vi "set_sensor_parameters_cluster.vi"(8 "error in (no error)":errorcluster, 9 "Sensor parameters":T1, 10 "Sensor number":u8, 11 "VISA resource name":refnum<visa-resource-name>) -> (0 "error out":errorcluster, 3 "VISA resource name out":refnum<visa-resource-name>)   [LabVIEW 2018]
doc: "Set the density of a material."
uses:
  Low Level/sensor_parameter_ring.ctl
  Low Level/sensor_parameters.ctl
panel:
  in  "Sensor parameter":T2 items=["Sensor Shutter Output", "Sensor Type", "Sensor Switch Output", "Auto-Z", "# of Positions", "# of Pulses", "Pulse On Time (s)", "Pulse Off Time (s)", "Recorder Output", "Recorder Function", "Recorder Range"]
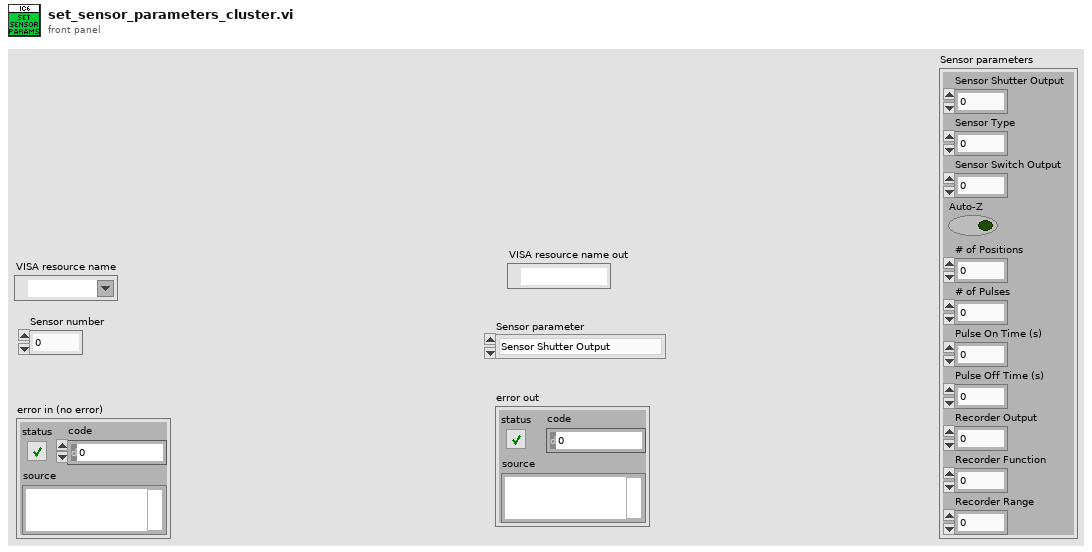
[diagram p1: front panel]
types:
  T1 = typedef "sensor_parameters.ctl" = cluster{"Sensor Shutter Output":u8, "Sensor Type":u8, "Sensor Switch Output":u8, "Auto-Z":bool, "# of Positions":u8, "# of Pulses":u8, "Pulse On Time (s)":sgl, "Pulse Off Time (s)":sgl, "Recorder Output":u8, "Recorder Function":u8, "Recorder Range":u32}
  T2 = typedef "sensor_parameter_ring.ctl" = u16
  T3 = typedef "LVStringsAndValuesArrayTypeDef_U16.ctl" = cluster{"String":string, "Value":u16}[]
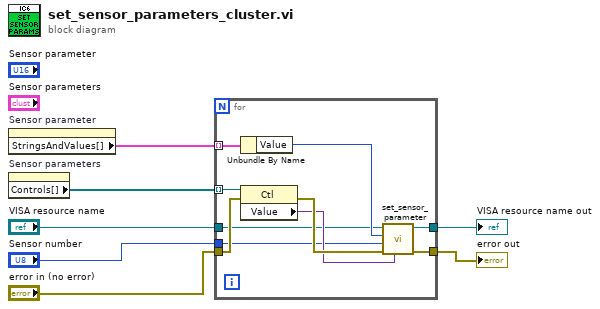
[diagram p0: block diagram]
diagram:
  n1 = property on="Sensor parameter" class="Ring (strict)"() -> ("StringsAndValues[]"=w3:T3)  [unwired: 2 in, 2 out]
  n2 = property on="Sensor parameters" class="Clust (strict)"() -> ("Controls[]"=w1:refnum<vi>[])  [unwired: 2 in, 2 out]
  n3 = for {
    tunnel: "VISA resource name" -> [w9]
    tunnel: [w13] -> w6
    tunnel: [w14] -> w2
    tunnel: "error in (no error)" -> [w16]
    tunnel: "Sensor number" -> [w8]
    tunnel: w3 -> [w12] mode=indexing
    tunnel: w1 -> [w17] mode=indexing
    n4 = Unbundle By Name(w12) -> ("Value"=w11:u16)
    n5 = property class="Ctl"(reference=w17, error in=w16) -> (error out=w15:errorcluster, "Value"=w10:variant)  [unwired: 1 out]
    n6 = call "set_sensor_parameter.vi"("Parameter"=w10, "error in (no error)"=w15, "Sensor number"=w8, "Sensor parameter"=w11, "VISA resource name"=w9) -> ("error out"=w14:errorcluster, "VISA resource name out"=w13:refnum<visa-resource-name>)  [unwired: 5 in]
  }
  "error out" <- w2
  "VISA resource name out" <- w6
